vi "Configure Trigger Source.vi"(8 "error in (no error)":errorcluster {"code" format="%.0x"}, 9 "Source (1: Software)":u16(ring)=1 items=["External", "Software", "Pin 1", "Pin 2", "Pin 3", "Transient 1", "Transient 2", "Transient 3", "Transient 4"], 10 "Channel Name (1)":string="1", 11 "VISA resource name":refnum<visa-resource-name>) -> (0 "error out":errorcluster {"code" format="%.0x"}, 3 "VISA resource name out":refnum<visa-resource-name>)   [LabVIEW 2010, in "Agilent N6700 Series.lvlib"]
doc: "Configures the trigger source the power supply waits for before changing the output signal. When the power supply receives a trigger signal on the source you specify, it changes its current limit and voltage level to the values of the agn6700>>Basic Operation>>Current Limit and agn6700>>Basic Operation>>Voltage Level properties, respectively."
uses:
  Agilent N6700 Series.lvlib
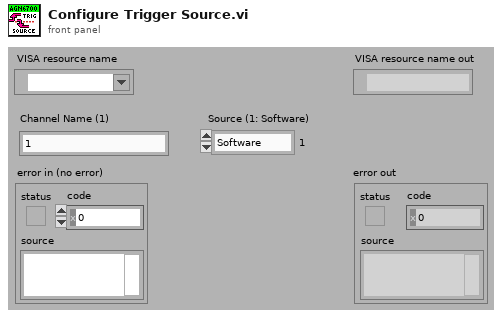
[diagram p1: front panel]
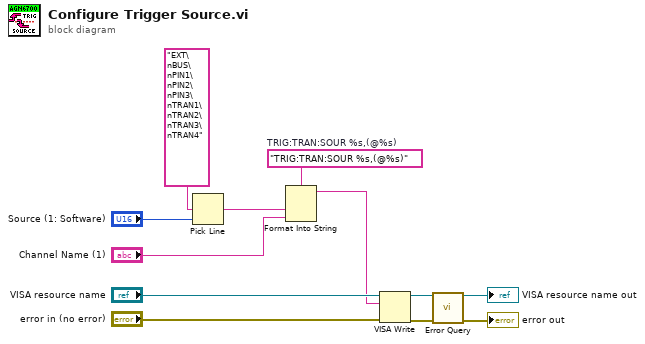
[diagram p0: block diagram]
diagram:
  w12 = "TRIG:TRAN:SOUR %s,(@%s)"  # TRIG:TRAN:SOUR %s,(@%s)
  n1 = Pick Line(multi-line string="EXT\nBUS\nPIN1\nPIN2\nPIN3\nTRAN1\nTRAN2\nTRAN3\nTRAN4", line index="Source (1: Software)") -> (output string=w8:string)  [unwired: 1 in]
  n2 = Format Into String(format string=w12, w8, "Channel Name (1)") -> (resulting string=w6:string)  [unwired: 2 in, 1 out]
  n3 = VISA Write(VISA resource name="VISA resource name", write buffer=w6, error in (no error)="error in (no error)") -> (VISA resource name out=w2:refnum<visa-resource-name>, error out=w1:errorcluster)  [unwired: 1 out]
  n4 = call "Error Query.vi"("VISA resource name"=w2, "error in (no error)"=w1) -> ("VISA resource name out"=→"VISA resource name out":refnum<visa-resource-name>, "error out"=→"error out":errorcluster)  [unwired: 10 in, 2 out]
